vi "Test VI.vi"() -> ()   [LabVIEW 2013]
uses:
  <vilib>/Utility/miscctls.llb/LVRectTypeDef.ctl
panel:
  in  "Top Level Tab Control":enum32{"<Module Name>"}(tab)
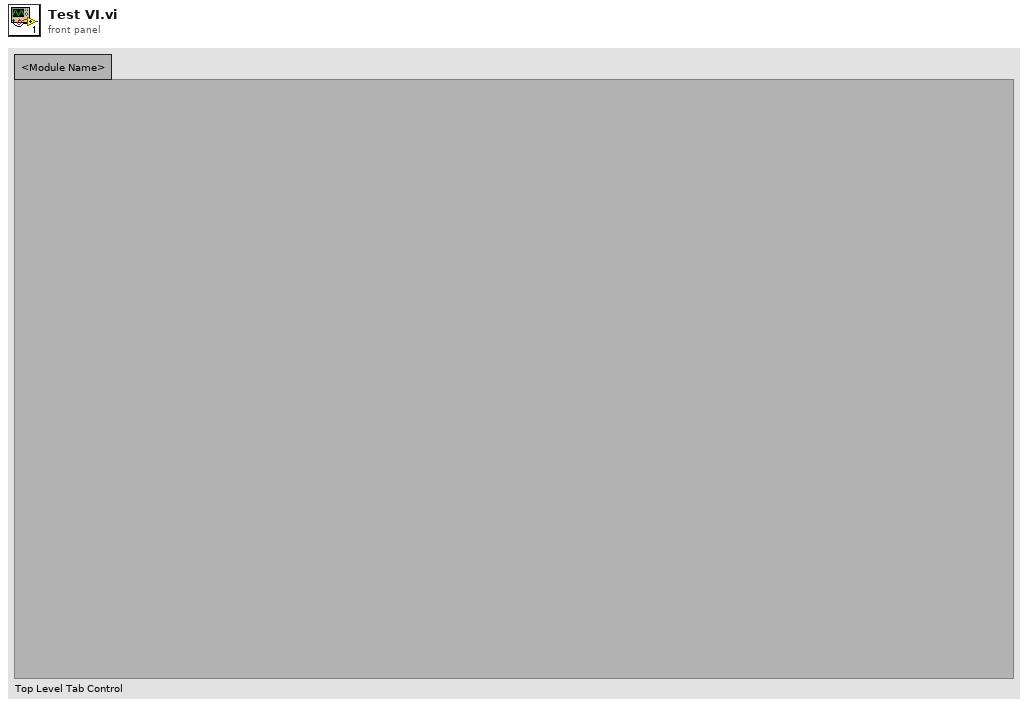
[diagram p1: front panel]
types:
  T1 = typedef "LVRectTypeDef.ctl" = cluster{"Left":i16, "Top":i16, "Right":i16, "Bottom":i16}
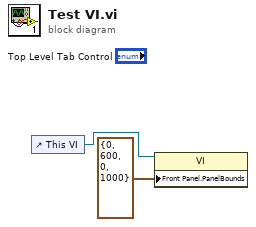
[diagram p0: block diagram]
diagram:
  n1 = control-ref of="This VI"() -> (w2:refnum<vi>)
  n2 = property class="VI"(reference=w2, "Front Panel.PanelBounds"=T1 {"Left"=0, "Top"=600, "Right"=0, "Bottom"=1000} ("Front Panel Window:Panel Bounds")) -> ()  [unwired: 1 in, 2 out]
